vi "UT_LV to TOML_002.vi"() -> ()   [LabVIEW 2017]
uses:
  <vilib>/addons/_JKI Toolkits/Caraya/classes/Assert/Assert True.vi
  <vilib>/addons/_JKI Toolkits/Caraya/classes/Assert/Assert Not Error.vi
  <vilib>/addons/_JKI Toolkits/Caraya/classes/Assert/Assert Error.vi
  <vilib>/addons/_JKI Toolkits/Caraya/classes/Test/Test.lvclass
  <vilib>/addons/_JKI Toolkits/Caraya/classes/Assert/Assert.lvclass
  lib/TOML.lvlib
panel:
  out "error out":errorcluster
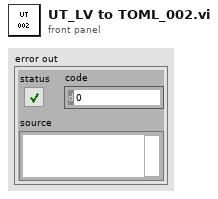
[diagram p1: front panel]
types:
  T1 = cluster{"cluster":cluster{"status":bool, "code":i32, "source":string, "error":errorcluster, "float-array":dbl[], "cluster-array":cluster{"nam":string, "value":dbl}[]}}
  T2 = cluster{"cluster":cluster{"status":bool, "cod":i32, "source":string, "error":errorcluster, "float-array":dbl[], "cluster-array":cluster{"name":string, "value":dbl}[]}}
  T3 = cluster{"status":bool, "code":i32, "source":string, "error":errorcluster, "float-array":dbl[], "cluster-array":cluster{"name":string, "value":dbl}[]}
  T4 = cluster{"cluster":cluster{"status":bool, "code":i32, "source":string, "error":errorcluster, "float-array":dbl[], "cluster-array":cluster{"name":string, "value":dbl}[]}}
  T5 = typedef "TOML.lvlib/TOML Value.ctl" = cluster{"type":enum16{"Table", "Array", "String", "Integer", "Float", "Boolean", "Offset Date-Time", "Local Date-Time", "Local Date", "Local Time"}, "value":variant}
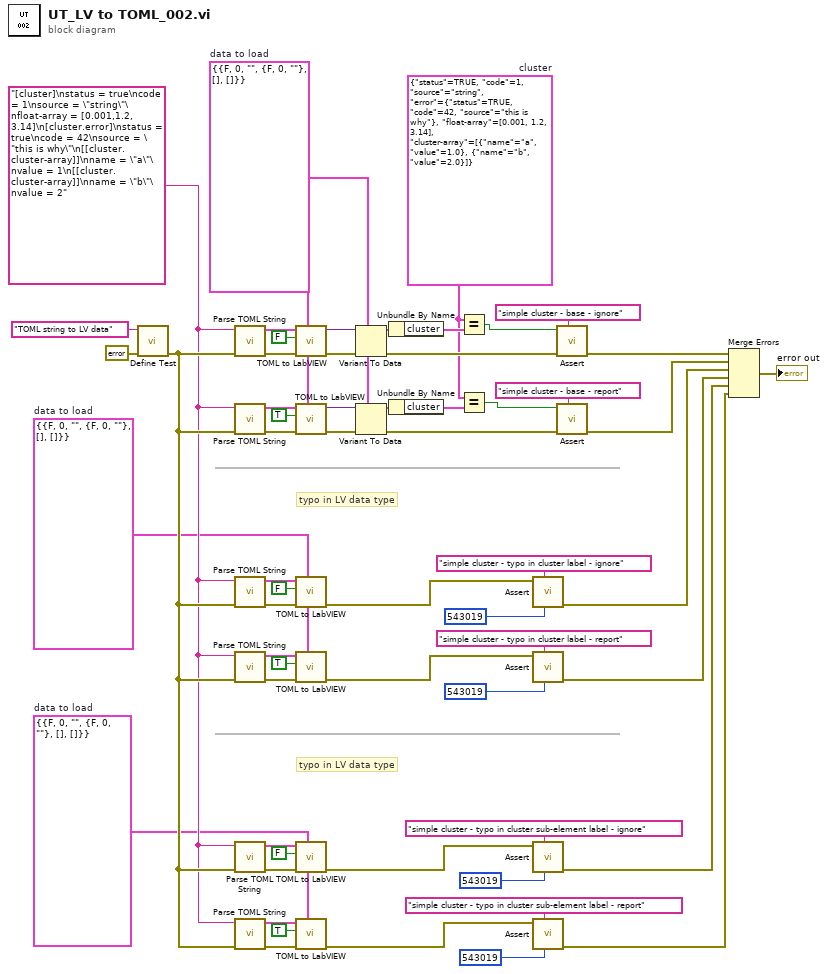
[diagram p0: block diagram]
diagram:
  w1 = T1 {"cluster"={"status"=FALSE, "code"=0, "source"="", "error"={"status"=FALSE, "code"=0, "source"=""}, "float-array"=[], "cluster-array"=[]}}  # data to load
  w2 = T2 {"cluster"={"status"=FALSE, "cod"=0, "source"="", "error"={"status"=FALSE, "code"=0, "source"=""}, "float-array"=[], "cluster-array"=[]}}  # data to load
  w3 = T3 {"status"=TRUE, "code"=1, "source"="string", "error"={"status"=TRUE, "code"=42, "source"="this is why"}, "float-array"=[0.001, 1.2, 3.14], "cluster-array"=[{"name"="a", "value"=1.0}, {"name"="b", "value"=2.0}]}  # cluster
  w4 = T4 {"cluster"={"status"=FALSE, "code"=0, "source"="", "error"={"status"=FALSE, "code"=0, "source"=""}, "float-array"=[], "cluster-array"=[]}}  # data to load
  w7 = "[cluster]\nstatus = true\ncode = 1\nsource = \"string\"\nfloat-array = [0.001,1.2, 3.14]\n[cluster.error]\nstatus = true\ncode = 42\nsource = \"this is why\"\n[[cluster.cluster-array]]\nname = \"a\"\nvalue = 1\n[[cluster.cluster-array]]\nname = \"b\"\nvalue = 2" ("String")
  # "typo in LV data type"
  # "typo in LV data type"
  n1 = call <vilib>:"Define Test.vi"("error in (no error)"=errorcluster {"status"=FALSE, "code"=0, "source"=""}, "Label (VI Title)"="TOML string to LV data") -> ("error out"=w8:errorcluster)  [unwired: 9 in]
  n2 = call "Parse TOML String.vi"("error in (no error)"=w8, "String"=w7) -> ("error out"=w55:errorcluster, "Value"=w54:T5)  [unwired: 8 in]
  n3 = call "Parse TOML String.vi"("error in (no error)"=w8, "String"=w7) -> ("error out"=w22:errorcluster, "Value"=w23:T5)  [unwired: 8 in]
  n4 = call "Parse TOML String.vi"("error in (no error)"=w8, "String"=w7) -> ("error out"=w45:errorcluster, "Value"=w46:T5)  [unwired: 8 in]
  n5 = call "Parse TOML String.vi"("error in (no error)"=w8, "String"=w7) -> ("error out"=w16:errorcluster, "Value"=w15:T5)  [unwired: 8 in]
  n6 = call "Parse TOML String.vi"("error in (no error)"=w8, "String"=w7) -> ("error out"=w39:errorcluster, "Value"=w38:T5)  [unwired: 8 in]
  n7 = call "Parse TOML String.vi"("error in (no error)"=w8, "String"=w7) -> ("error out"=w11:errorcluster, "Value"=w12:T5)  [unwired: 8 in]
  n8 = call "TOML to LabVIEW.vi"("Default Value"=w4, "error in (no error)"=w55, "Error if missing element"=FALSE, "TOML Value"=w54) -> ("error out"=w53:errorcluster, "LV Value"=w51:variant)  [unwired: 6 in]
  n9 = call "TOML to LabVIEW.vi"("Default Value"=w4, "error in (no error)"=w22, "Error if missing element"=TRUE, "TOML Value"=w23) -> ("error out"=w26:errorcluster, "LV Value"=w28:variant)  [unwired: 6 in]
  n10 = call "TOML to LabVIEW.vi"("Default Value"=w2, "error in (no error)"=w45, "Error if missing element"=FALSE, "TOML Value"=w46) -> ("error out"=w42:errorcluster)  [unwired: 6 in, 1 out]
  n11 = call "TOML to LabVIEW.vi"("Default Value"=w2, "error in (no error)"=w16, "Error if missing element"=TRUE, "TOML Value"=w15) -> ("error out"=w18:errorcluster)  [unwired: 6 in, 1 out]
  n12 = call "TOML to LabVIEW.vi"("Default Value"=w1, "error in (no error)"=w39, "Error if missing element"=FALSE, "TOML Value"=w38) -> ("error out"=w41:errorcluster)  [unwired: 6 in, 1 out]
  n13 = call "TOML to LabVIEW.vi"("Default Value"=w1, "error in (no error)"=w11, "Error if missing element"=TRUE, "TOML Value"=w12) -> ("error out"=w9:errorcluster)  [unwired: 6 in, 1 out]
  n14 = Variant To Data(error in=w53, type=w4, Variant=w51) -> (data=w50:T4, error out=w52:errorcluster)
  n15 = Variant To Data(error in=w26, type=w4, Variant=w28) -> (data=w29:T4, error out=w27:errorcluster)
  n16 = Unbundle By Name(w50) -> ("cluster"=w47:T3)
  n17 = Unbundle By Name(w29) -> ("cluster"=w31:T3)
  n18 = Equal?(x=w3, y=w47) -> (x = y?=w49:bool)
  n19 = Equal?(x=w3, y=w31) -> (x = y?=w30:bool)
  n20 = call-poly <vilib>:"Assert.vi"("error code (1)"=543019, "Label"="simple cluster - typo in cluster label - ignore" ("Label (VI Title)"), "Not Error?"=w42) -> ("error out"=w43:errorcluster)  [unwired: 8 in]
  n21 = call-poly <vilib>:"Assert.vi"("error code (1)"=543019, "Label"="simple cluster - typo in cluster label - report" ("Label (VI Title)"), "Error?"=w18) -> ("error out"=w5:errorcluster)  [unwired: 8 in]
  n22 = call-poly <vilib>:"Assert.vi"("error code (1)"=543019, "Label"="simple cluster - typo in cluster sub-element label - ignore" ("Label (VI Title)"), "Not Error?"=w41) -> ("error out"=w37:errorcluster)  [unwired: 8 in]
  n23 = call-poly <vilib>:"Assert.vi"("error code (1)"=543019, "Label"="simple cluster - typo in cluster sub-element label - report" ("Label (VI Title)"), "Error?"=w9) -> ("error out"=w6:errorcluster)  [unwired: 8 in]
  n24 = call-poly <vilib>:"Assert.vi"("Label"="simple cluster - base - ignore" ("Label (VI Title)"), "error in (no error)"=w52, "True?"=w49) -> ("error out"=w58:errorcluster)  [unwired: 8 in]
  n25 = call-poly <vilib>:"Assert.vi"("Label"="simple cluster - base - report" ("Label (VI Title)"), "error in (no error)"=w27, "True?"=w30) -> ("error out"=w21:errorcluster)  [unwired: 8 in]
  n26 = Merge Errors(w58, w21, w43, w5, w37, w6) -> (→"error out":errorcluster)
